vi "SetAppMetadata.vi"(8 "No Error":errorcluster, 9 "App Identifier":string, 10 "App Version":string, 11 "App Name":string) -> (0 "error out":errorcluster)   [LabVIEW 2026, in "SDL3.lvlib" / "Init.lvlib"]
doc: "<B>Summary</B>\nSpecify basic metadata about your app.\n\n<B>Remarks</B>\nYou can optionally provide metadata about your app to SDL. This is not required, but strongly encouraged.\n\nThere are several locations where SDL can make use of metadata (an \"About\" box in the macOS menu bar, the name of the app can be shown on some audio mixers, etc). Any piece of metadata can be left as NULL, if a specific detail doesn't make sense for the app.\n\nThis function should be called as early as possible, before <B>SDL_Init</B>. Multiple calls to this function are allowed, but various state might not change once it has been set up with a previous call to this function.\n\nThis is a simplified interface for the most important information. You can supply significantly more detailed metadata with <B>SDL_SetAppMetadataProperty()</B>."
uses:
  Init.lvlib
  <vilib>/Utility/error.llb/Error Cluster From Error Code.vi
  Error/Error.lvlib
  Lib/SDL3.dll
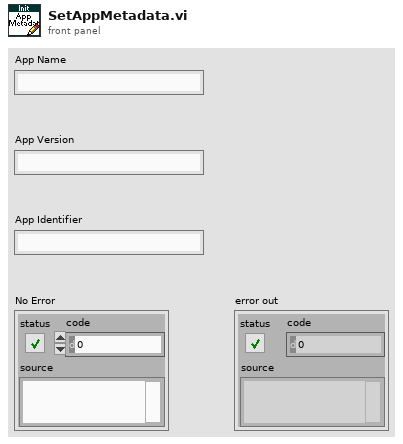
[diagram p1: front panel]
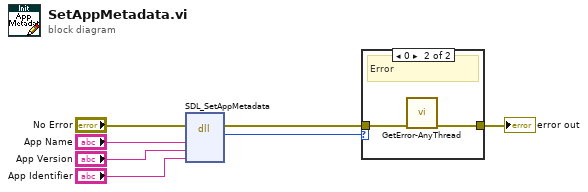
[diagram p0: block diagram]
diagram:
  n1 = dll-call lib="C:/Users/saukko/Dev/LV-SDL3/Sources/SDL3/Lib/SDL3.*" fn="SDL_SetAppMetadata"(error in="No Error", "appname"="App Name", "appversion"="App Version", "appidentifier"="App Identifier") -> (error out=w4:errorcluster, "return type"=w5:i32)  [unwired: 5 in, 1 out]
  n2 = case shown="0" w5 {
    tunnel: w4 -> [w8 w10]
    tunnel: [w8 w9] -> w6
    frame Default {
      # "Ok"
    }
    frame 0 {
      # "Error"
      n3 = call "GetError-AnyThread.vi"("No Error"=w10) -> ("Error Out"=w9:errorcluster)  [unwired: 10 in]
    }
  }
  "error out" <- w6
